vi "Char pro.vi"() -> ()   [LabVIEW 2010]
panel:
  in  "stop":bool
  out "Perreo Intenso":bool
  out "Tranqui":bool
  out "Morido":bool
  out "Temperatura":dbl(slide) scale=0.0..100.0
  in  "Velocidad en seundos":dbl(knob) scale=0.0..1.0
  out "Waveform Chart":dbl(graph)
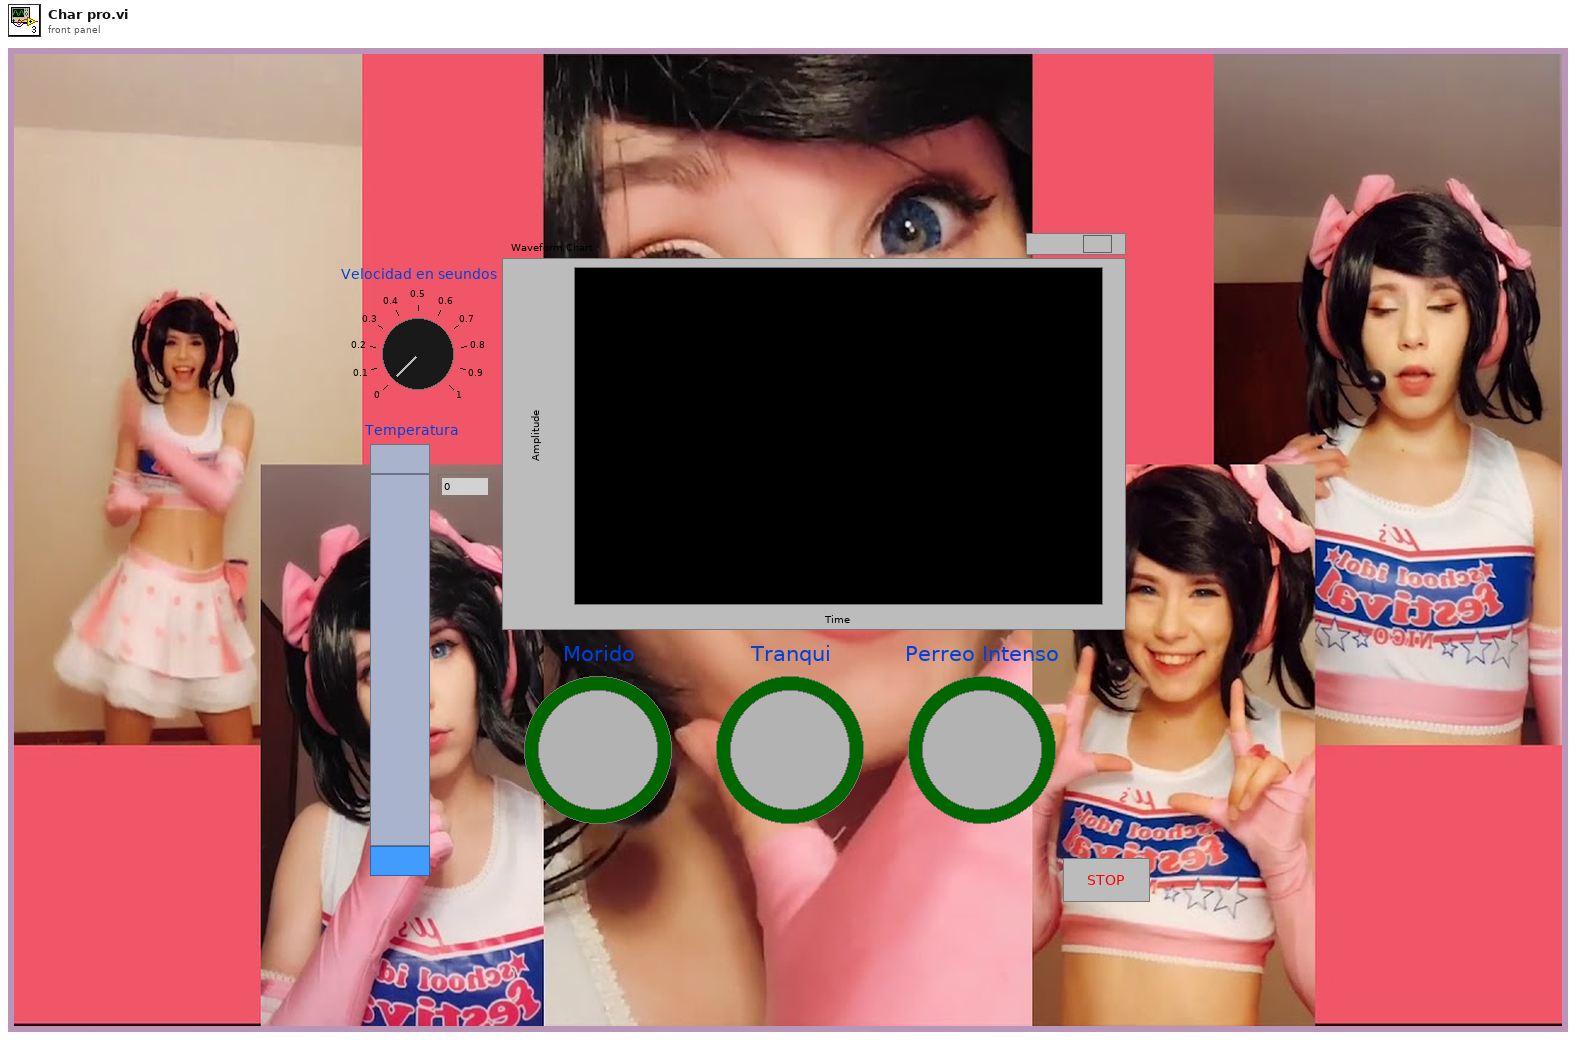
[diagram p1: front panel]
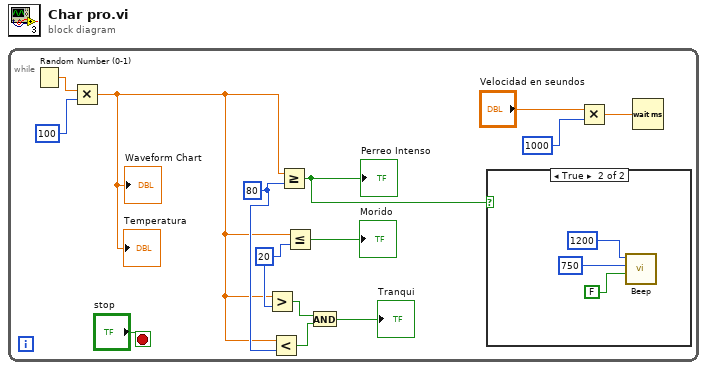
[diagram p0: block diagram]
diagram:
  n1 = while {
    stop <- "stop" stop-if-true
    w7 = 20
    w6 = 80
    n2 = Random Number (0-1)() -> (number: 0 to 1=w13:dbl)
    n3 = Multiply(x=w13, y=100) -> (x*y=w1:dbl)
    "Waveform Chart" <- w1
    "Temperatura" <- w1
    n4 = Greater?(x=w1, y=w7) -> (0:w5:bool)
    n5 = Less?(x=w1, y=w6) -> (x < y?=w4:bool)
    n6 = Greater Or Equal?(x=w1, y=w6) -> (x >= y?=w2:bool)
    "Perreo Intenso" <- w2
    n7 = Less Or Equal?(x=w1, y=w7) -> (x <= y?=→"Morido":bool)
    n8 = And(x=w5, y=w4) -> (x .and. y?=→"Tranqui":bool)
    n9 = case shown="True" w2 {
      frame False {
      }
      frame True {
        n10 = call <vilib>:"Beep.vi"("use system alert? (T)"=FALSE, "duration (msec)"=750, "frequency (Hz)"=1200) -> ()  [unwired: 9 in]
      }
    }
    n11 = Multiply(x="Velocidad en seundos", y=1000) -> (x*y=w9:dbl)
    n12 = Wait (ms)(milliseconds to wait=w9) -> ()  [unwired: 1 out]
  }
